vi "Parallel Executing Test Code.vi"(9 "Test Complete Event":refnum<user-event>, 10 "Positions":u32[](array[numeric]), 11 "RF PostFlash in":refnum<class "RF PostFlash.lvclass">) -> ()   [LabVIEW 2015, in "RF PostFlash.lvclass"]
uses:
  RF PostFlash.lvclass
  Common RF Tests/RF Common Tests.lvclass
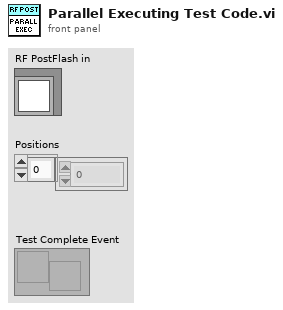
[diagram p1: front panel]
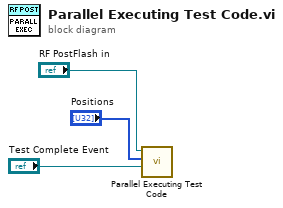
[diagram p0: block diagram]
diagram:
  n1 = call-parent "Parallel Executing Test Code.vi"("Test Complete Event"="Test Complete Event", "Positions"="Positions", "Parallel Test in"="RF PostFlash in") -> ()  [unwired: 9 in]
